vi "FRCts20_Backend_INI_Save.vi"(8 "error in (no error)":errorcluster, 10 "Save? (T)":bool=TRUE, 11 "INI Controller in":refnum<class "FRCts20_Backend_INI Controller.lvclass">) -> (0 "error out":errorcluster, 3 "INI Controller out":refnum<class "FRCts20_Backend_INI Controller.lvclass">)   [LabVIEW 2014, in "FRCts20_Backend_Engine.lvlib" / "FRCts20_Backend_INI Controller.lvclass"]
uses:
  FRCts20_Backend_INI Controller.lvclass
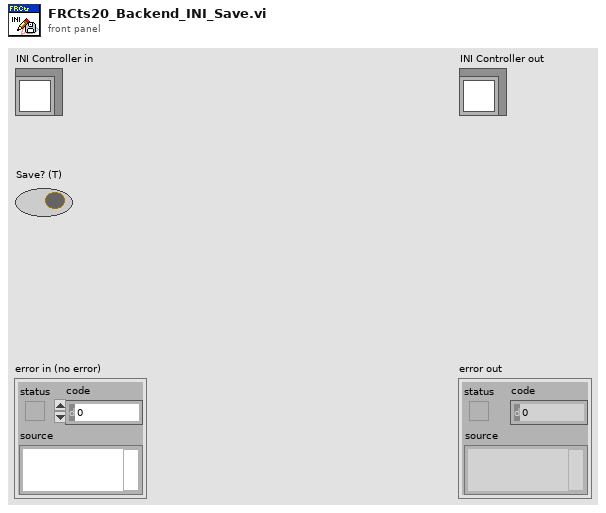
[diagram p1: front panel]
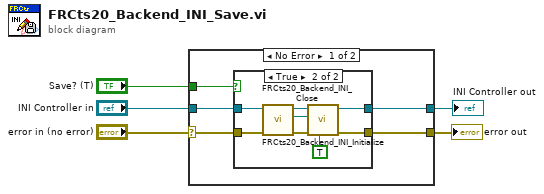
[diagram p0: block diagram]
diagram:
  n1 = case shown="No Error" "error in (no error)" {
    selector: "error in (no error)" -> [w7 w22]
    tunnel: [w9 w22] -> w4
    tunnel: [w10 w21] -> w2
    tunnel: "INI Controller in" -> [w8 w21]
    tunnel: "Save? (T)" -> [w6 _]
    frame No Error {
      n2 = case shown="True" w6 {
        tunnel: [w12 w20] -> w10
        tunnel: [w11 w19] -> w9
        tunnel: w8 -> [w12 w18]
        tunnel: w7 -> [w11 w13]
        frame False {
        }
        frame True {
          n3 = call "FRCts20_Backend_INI_Close.vi"("error in (no error)"=w13, "INI Controller in"=w18) -> ("error out"=w15:errorcluster, "file path"=w16:path, "INI Controller out"=w17:refnum<class "FRCts20_Backend_INI Controller.lvclass">)  [unwired: 7 in]
          n4 = call "FRCts20_Backend_INI_Initialize.vi"("Inhibit (F)"=TRUE ("Inhibit"), "error in (no error)"=w15, "Config Path"=w16, "INI Controller in"=w17) -> ("error out"=w19:errorcluster, "INI Controller out"=w20:refnum<class "FRCts20_Backend_INI Controller.lvclass">)  [unwired: 6 in]
        }
      }
    }
    frame Error {
    }
  }
  "error out" <- w4
  "INI Controller out" <- w2
